vi "GenerareDateCifre.vi"() -> (0 "path":path)   [LabVIEW 2025]
uses:
  <vilib>/National Instruments/NI Super Simple Neural Networks/Types/Teaching Vector.ctl
  <vilib>/National Instruments/NI Super Simple Neural Networks/Types/1D Array.ctl
  <vilib>/National Instruments/NI Super Simple Neural Networks/Neural Network.lvclass
panel:
  out "error out":errorcluster
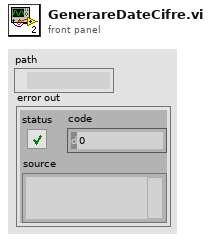
[diagram p1: front panel]
types:
  T1 = typedef "Neural Network.lvclass/Teaching Vector.ctl" = cluster{"Inputs":T2, "Expected Outputs":T2}
  T2 = typedef "Neural Network.lvclass/1D Array.ctl" = cluster{"1D Array":dbl[]}
  T3 = enum16{"open", "replace", "create", "open or create", "replace or create", "replace or create with confirmation"}
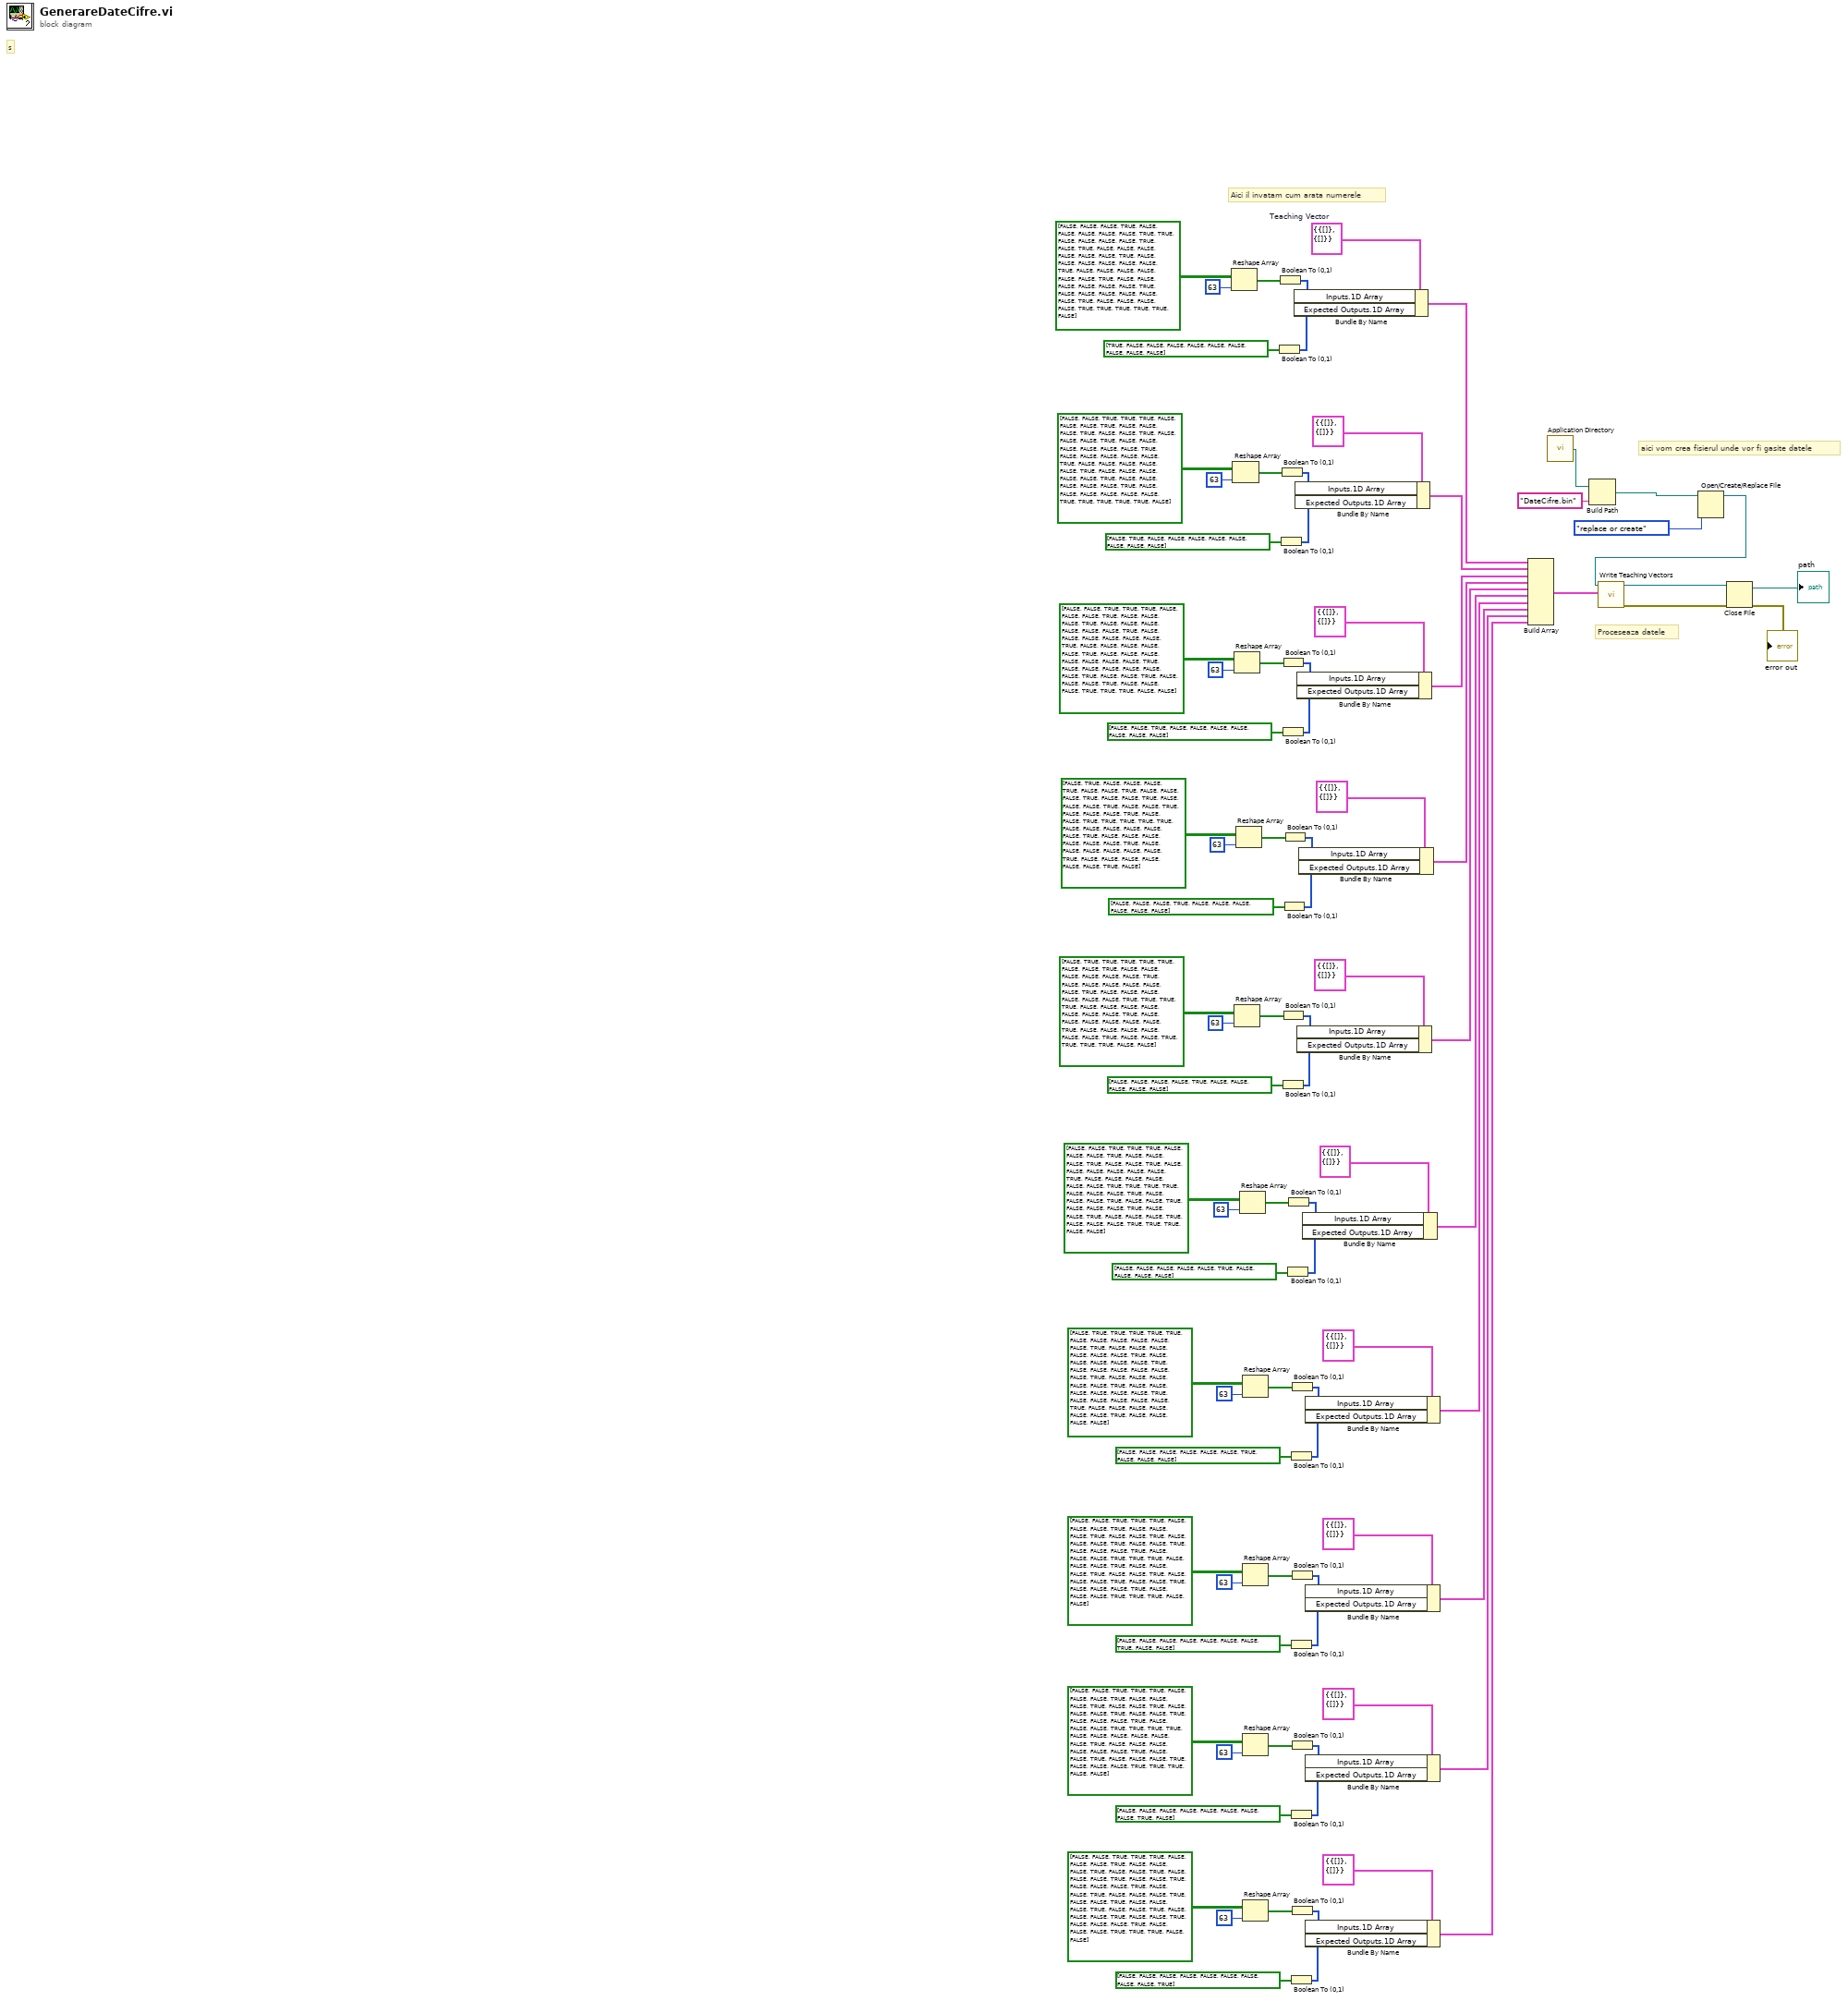
[diagram p0: block diagram]
diagram:
  w86 = T1 {"Inputs"={"1D Array"=[]}, "Expected Outputs"={"1D Array"=[]}}  # Teaching Vector
  # "s"
  # "Proceseaza datele"
  # "aici vom crea fisierul unde vor fi gasite datele"
  # "Aici il invatam cum arata numerele"
  n1 = Reshape Array(bool[][] [[FALSE, FALSE, FALSE, TRUE, FALSE, FALSE, FALSE], [FALSE, FALSE, TRUE, TRUE, FALSE, FALSE, FALSE], [FALSE, TRUE, FALSE, TRUE, FALSE, FALSE, FALSE], [FALSE, FALSE, FALSE, TRUE, FALSE, FALSE, FALSE], [FALSE, FALSE, FALSE, TRUE, FALSE, FALSE, FALSE], [FALSE, FALSE, FALSE, TRUE, FALSE, FALSE, FALSE], [FALSE, FALSE, FALSE, TRUE, FALSE, FALSE, FALSE], [FALSE, FALSE, FALSE, TRUE, FALSE, FALSE, FALSE], [FALSE, TRUE, TRUE, TRUE, TRUE, TRUE, FALSE]], 63 ("dimension size")) -> (w88:bool[])
  n2 = Reshape Array(bool[][] [[FALSE, FALSE, TRUE, TRUE, TRUE, FALSE, FALSE], [FALSE, TRUE, FALSE, FALSE, FALSE, TRUE, FALSE], [FALSE, TRUE, FALSE, FALSE, FALSE, TRUE, FALSE], [FALSE, FALSE, FALSE, FALSE, FALSE, TRUE, FALSE], [FALSE, FALSE, FALSE, FALSE, TRUE, FALSE, FALSE], [FALSE, FALSE, FALSE, TRUE, FALSE, FALSE, FALSE], [FALSE, FALSE, TRUE, FALSE, FALSE, FALSE, FALSE], [FALSE, TRUE, FALSE, FALSE, FALSE, FALSE, FALSE], [FALSE, TRUE, TRUE, TRUE, TRUE, TRUE, FALSE]], 63 ("dimension size")) -> (w70:bool[])
  n3 = Reshape Array(bool[][] [[FALSE, FALSE, TRUE, TRUE, TRUE, FALSE, FALSE], [FALSE, TRUE, FALSE, FALSE, FALSE, TRUE, FALSE], [FALSE, FALSE, FALSE, FALSE, FALSE, TRUE, FALSE], [FALSE, FALSE, FALSE, FALSE, FALSE, TRUE, FALSE], [FALSE, FALSE, FALSE, FALSE, TRUE, FALSE, FALSE], [FALSE, FALSE, FALSE, FALSE, FALSE, TRUE, FALSE], [FALSE, FALSE, FALSE, FALSE, FALSE, TRUE, FALSE], [FALSE, TRUE, FALSE, FALSE, FALSE, TRUE, FALSE], [FALSE, FALSE, TRUE, TRUE, TRUE, FALSE, FALSE]], 63 ("dimension size")) -> (w63:bool[])
  n4 = Reshape Array(bool[][] [[FALSE, TRUE, TRUE, TRUE, TRUE, TRUE, FALSE], [FALSE, TRUE, FALSE, FALSE, FALSE, FALSE, FALSE], [FALSE, TRUE, FALSE, FALSE, FALSE, FALSE, FALSE], [FALSE, TRUE, FALSE, FALSE, FALSE, FALSE, FALSE], [FALSE, TRUE, TRUE, TRUE, TRUE, FALSE, FALSE], [FALSE, FALSE, FALSE, FALSE, FALSE, TRUE, FALSE], [FALSE, FALSE, FALSE, FALSE, FALSE, TRUE, FALSE], [FALSE, FALSE, FALSE, FALSE, FALSE, TRUE, FALSE], [FALSE, TRUE, TRUE, TRUE, TRUE, FALSE, FALSE]], 63 ("dimension size")) -> (w49:bool[])
  n5 = Reshape Array(bool[][] [[FALSE, TRUE, FALSE, FALSE, FALSE, TRUE, FALSE], [FALSE, TRUE, FALSE, FALSE, FALSE, TRUE, FALSE], [FALSE, TRUE, FALSE, FALSE, FALSE, TRUE, FALSE], [FALSE, TRUE, FALSE, FALSE, FALSE, TRUE, FALSE], [FALSE, TRUE, TRUE, TRUE, TRUE, TRUE, FALSE], [FALSE, FALSE, FALSE, FALSE, FALSE, TRUE, FALSE], [FALSE, FALSE, FALSE, FALSE, FALSE, TRUE, FALSE], [FALSE, FALSE, FALSE, FALSE, FALSE, TRUE, FALSE], [FALSE, FALSE, FALSE, FALSE, FALSE, TRUE, FALSE]], 63 ("dimension size")) -> (w56:bool[])
  n6 = Reshape Array(bool[][] [[FALSE, FALSE, TRUE, TRUE, TRUE, FALSE, FALSE], [FALSE, TRUE, FALSE, FALSE, FALSE, TRUE, FALSE], [FALSE, TRUE, FALSE, FALSE, FALSE, FALSE, FALSE], [FALSE, TRUE, FALSE, FALSE, FALSE, FALSE, FALSE], [FALSE, TRUE, TRUE, TRUE, TRUE, FALSE, FALSE], [FALSE, TRUE, FALSE, FALSE, FALSE, TRUE, FALSE], [FALSE, TRUE, FALSE, FALSE, FALSE, TRUE, FALSE], [FALSE, TRUE, FALSE, FALSE, FALSE, TRUE, FALSE], [FALSE, FALSE, TRUE, TRUE, TRUE, FALSE, FALSE]], 63 ("dimension size")) -> (w42:bool[])
  n7 = Reshape Array(bool[][] [[FALSE, TRUE, TRUE, TRUE, TRUE, TRUE, FALSE], [FALSE, FALSE, FALSE, FALSE, FALSE, TRUE, FALSE], [FALSE, FALSE, FALSE, FALSE, FALSE, TRUE, FALSE], [FALSE, FALSE, FALSE, FALSE, TRUE, FALSE, FALSE], [FALSE, FALSE, FALSE, FALSE, TRUE, FALSE, FALSE], [FALSE, FALSE, FALSE, TRUE, FALSE, FALSE, FALSE], [FALSE, FALSE, FALSE, TRUE, FALSE, FALSE, FALSE], [FALSE, FALSE, TRUE, FALSE, FALSE, FALSE, FALSE], [FALSE, FALSE, TRUE, FALSE, FALSE, FALSE, FALSE]], 63 ("dimension size")) -> (w35:bool[])
  n8 = Reshape Array(bool[][] [[FALSE, FALSE, TRUE, TRUE, TRUE, FALSE, FALSE], [FALSE, TRUE, FALSE, FALSE, FALSE, TRUE, FALSE], [FALSE, TRUE, FALSE, FALSE, FALSE, TRUE, FALSE], [FALSE, TRUE, FALSE, FALSE, FALSE, TRUE, FALSE], [FALSE, FALSE, TRUE, TRUE, TRUE, FALSE, FALSE], [FALSE, TRUE, FALSE, FALSE, FALSE, TRUE, FALSE], [FALSE, TRUE, FALSE, FALSE, FALSE, TRUE, FALSE], [FALSE, TRUE, FALSE, FALSE, FALSE, TRUE, FALSE], [FALSE, FALSE, TRUE, TRUE, TRUE, FALSE, FALSE]], 63 ("dimension size")) -> (w28:bool[])
  n9 = Reshape Array(bool[][] [[FALSE, FALSE, TRUE, TRUE, TRUE, FALSE, FALSE], [FALSE, TRUE, FALSE, FALSE, FALSE, TRUE, FALSE], [FALSE, TRUE, FALSE, FALSE, FALSE, TRUE, FALSE], [FALSE, TRUE, FALSE, FALSE, FALSE, TRUE, FALSE], [FALSE, FALSE, TRUE, TRUE, TRUE, TRUE, FALSE], [FALSE, FALSE, FALSE, FALSE, FALSE, TRUE, FALSE], [FALSE, FALSE, FALSE, FALSE, FALSE, TRUE, FALSE], [FALSE, TRUE, FALSE, FALSE, FALSE, TRUE, FALSE], [FALSE, FALSE, TRUE, TRUE, TRUE, FALSE, FALSE]], 63 ("dimension size")) -> (w21:bool[])
  n10 = Reshape Array(bool[][] [[FALSE, FALSE, TRUE, TRUE, TRUE, FALSE, FALSE], [FALSE, TRUE, FALSE, FALSE, FALSE, TRUE, FALSE], [FALSE, TRUE, FALSE, FALSE, FALSE, TRUE, FALSE], [FALSE, TRUE, FALSE, FALSE, FALSE, TRUE, FALSE], [FALSE, TRUE, FALSE, FALSE, FALSE, TRUE, FALSE], [FALSE, TRUE, FALSE, FALSE, FALSE, TRUE, FALSE], [FALSE, TRUE, FALSE, FALSE, FALSE, TRUE, FALSE], [FALSE, TRUE, FALSE, FALSE, FALSE, TRUE, FALSE], [FALSE, FALSE, TRUE, TRUE, TRUE, FALSE, FALSE]], 63 ("dimension size")) -> (w14:bool[])
  n11 = Boolean To (0,1)(Boolean=bool[] [TRUE, FALSE, FALSE, FALSE, FALSE, FALSE, FALSE, FALSE, FALSE, FALSE]) -> (0, 1=w84:i16[])
  n12 = Boolean To (0,1)(Boolean=w88) -> (0, 1=w85:i16[])
  n13 = Boolean To (0,1)(Boolean=bool[] [FALSE, TRUE, FALSE, FALSE, FALSE, FALSE, FALSE, FALSE, FALSE, FALSE]) -> (0, 1=w66:i16[])
  n14 = Boolean To (0,1)(Boolean=w70) -> (0, 1=w67:i16[])
  n15 = Boolean To (0,1)(Boolean=bool[] [FALSE, FALSE, TRUE, FALSE, FALSE, FALSE, FALSE, FALSE, FALSE, FALSE]) -> (0, 1=w59:i16[])
  n16 = Boolean To (0,1)(Boolean=bool[] [FALSE, FALSE, FALSE, FALSE, TRUE, FALSE, FALSE, FALSE, FALSE, FALSE]) -> (0, 1=w45:i16[])
  n17 = Boolean To (0,1)(Boolean=w63) -> (0, 1=w60:i16[])
  n18 = Boolean To (0,1)(Boolean=w49) -> (0, 1=w46:i16[])
  n19 = Boolean To (0,1)(Boolean=bool[] [FALSE, FALSE, FALSE, TRUE, FALSE, FALSE, FALSE, FALSE, FALSE, FALSE]) -> (0, 1=w52:i16[])
  n20 = Boolean To (0,1)(Boolean=w56) -> (0, 1=w53:i16[])
  n21 = Boolean To (0,1)(Boolean=bool[] [FALSE, FALSE, FALSE, FALSE, FALSE, TRUE, FALSE, FALSE, FALSE, FALSE]) -> (0, 1=w38:i16[])
  n22 = Boolean To (0,1)(Boolean=w42) -> (0, 1=w39:i16[])
  n23 = Boolean To (0,1)(Boolean=bool[] [FALSE, FALSE, FALSE, FALSE, FALSE, FALSE, TRUE, FALSE, FALSE, FALSE]) -> (0, 1=w31:i16[])
  n24 = Boolean To (0,1)(Boolean=bool[] [FALSE, FALSE, FALSE, FALSE, FALSE, FALSE, FALSE, TRUE, FALSE, FALSE]) -> (0, 1=w24:i16[])
  n25 = Boolean To (0,1)(Boolean=bool[] [FALSE, FALSE, FALSE, FALSE, FALSE, FALSE, FALSE, FALSE, TRUE, FALSE]) -> (0, 1=w17:i16[])
  n26 = Boolean To (0,1)(Boolean=bool[] [FALSE, FALSE, FALSE, FALSE, FALSE, FALSE, FALSE, FALSE, FALSE, TRUE]) -> (0, 1=w10:i16[])
  n27 = Boolean To (0,1)(Boolean=w35) -> (0, 1=w32:i16[])
  n28 = Boolean To (0,1)(Boolean=w28) -> (0, 1=w25:i16[])
  n29 = Boolean To (0,1)(Boolean=w21) -> (0, 1=w18:i16[])
  n30 = Boolean To (0,1)(Boolean=w14) -> (0, 1=w11:i16[])
  n31 = Bundle By Name "Bundle By Name"(cluster=w86, "Inputs.1D Array"=w85, "Expected Outputs.1D Array"=w84) -> (w83:T1)
  n32 = Bundle By Name(cluster=T1 {"Inputs"={"1D Array"=[]}, "Expected Outputs"={"1D Array"=[]}} ("Teaching Vector"), "Inputs.1D Array"=w67, "Expected Outputs.1D Array"=w66) -> (w9:T1)
  n33 = Bundle By Name(cluster=T1 {"Inputs"={"1D Array"=[]}, "Expected Outputs"={"1D Array"=[]}} ("Teaching Vector"), "Inputs.1D Array"=w60, "Expected Outputs.1D Array"=w59) -> (w8:T1)
  n34 = Bundle By Name(cluster=T1 {"Inputs"={"1D Array"=[]}, "Expected Outputs"={"1D Array"=[]}} ("Teaching Vector"), "Inputs.1D Array"=w46, "Expected Outputs.1D Array"=w45) -> (w6:T1)
  n35 = Bundle By Name(cluster=T1 {"Inputs"={"1D Array"=[]}, "Expected Outputs"={"1D Array"=[]}} ("Teaching Vector"), "Inputs.1D Array"=w53, "Expected Outputs.1D Array"=w52) -> (w7:T1)
  n36 = Bundle By Name(cluster=T1 {"Inputs"={"1D Array"=[]}, "Expected Outputs"={"1D Array"=[]}} ("Teaching Vector"), "Inputs.1D Array"=w39, "Expected Outputs.1D Array"=w38) -> (w5:T1)
  n37 = Bundle By Name(cluster=T1 {"Inputs"={"1D Array"=[]}, "Expected Outputs"={"1D Array"=[]}} ("Teaching Vector"), "Inputs.1D Array"=w32, "Expected Outputs.1D Array"=w31) -> (w4:T1)
  n38 = Bundle By Name(cluster=T1 {"Inputs"={"1D Array"=[]}, "Expected Outputs"={"1D Array"=[]}} ("Teaching Vector"), "Inputs.1D Array"=w25, "Expected Outputs.1D Array"=w24) -> (w3:T1)
  n39 = Bundle By Name(cluster=T1 {"Inputs"={"1D Array"=[]}, "Expected Outputs"={"1D Array"=[]}} ("Teaching Vector"), "Inputs.1D Array"=w18, "Expected Outputs.1D Array"=w17) -> (w2:T1)
  n40 = Bundle By Name(cluster=T1 {"Inputs"={"1D Array"=[]}, "Expected Outputs"={"1D Array"=[]}} ("Teaching Vector"), "Inputs.1D Array"=w11, "Expected Outputs.1D Array"=w10) -> (w1:T1)
  n41 = Build Array "Build Array"(w83, w9, w8, w7, w6, w5, w4, w3, w2, w1) -> (w82:T1[])
  n42 = call <vilib>:"Application Directory.vi"() -> ("Application Directory"=w81:path)
  n43 = Build Path(base path=w81, name or relative path="DateCifre.bin") -> (appended path=w79:path)
  n44 = Open/Create/Replace File(file path (use dialog)=w79, operation (0:open)=T3."replace or create") -> (refnum out=w77:refnum<file>)  [unwired: 4 in, 2 out]
  n45 = call <vilib>:"Write Teaching Vectors.vi"("Teaching Vectors"=w82, "Teaching File Ref In"=w77) -> ("Error Out"=w75:errorcluster, "Teaching File Ref Out"=w76:refnum<file>)  [unwired: 8 in]
  n46 = Close File(refnum=w76, error in=w75) -> (path=→"path":path, error out=→"error out":errorcluster)
